vi "benchmarks_fileSHA1.vi"() -> ()   [LabVIEW 2013]
uses:
  SHA-1/SHA-1.lvclass
  <vilib>/Analysis/baseanly.llb/Mean (DBL).vi
  SHA-1/Enqueue File.vi
  SHA-1/pad.vi
  <vilib>/Analysis/NI_AALBase.lvlib
  SHA-1/SHA-1.lvlib
panel:
  out "MISSING ALGORITHM":bool
  out "equal hashes":bool
  out "% gain":dbl
  out "LVOS":dbl
  out "Other Algo":dbl
  in  "filepath":path
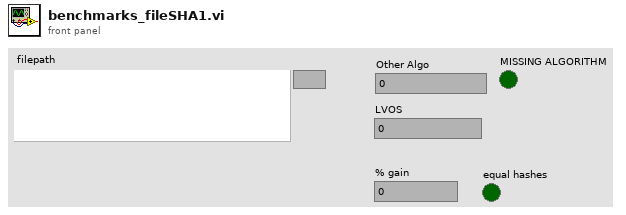
[diagram p1: front panel]
types:
  T1 = enum16{"open", "replace", "create", "open or create", "replace or create", "replace or create with confirmation"}
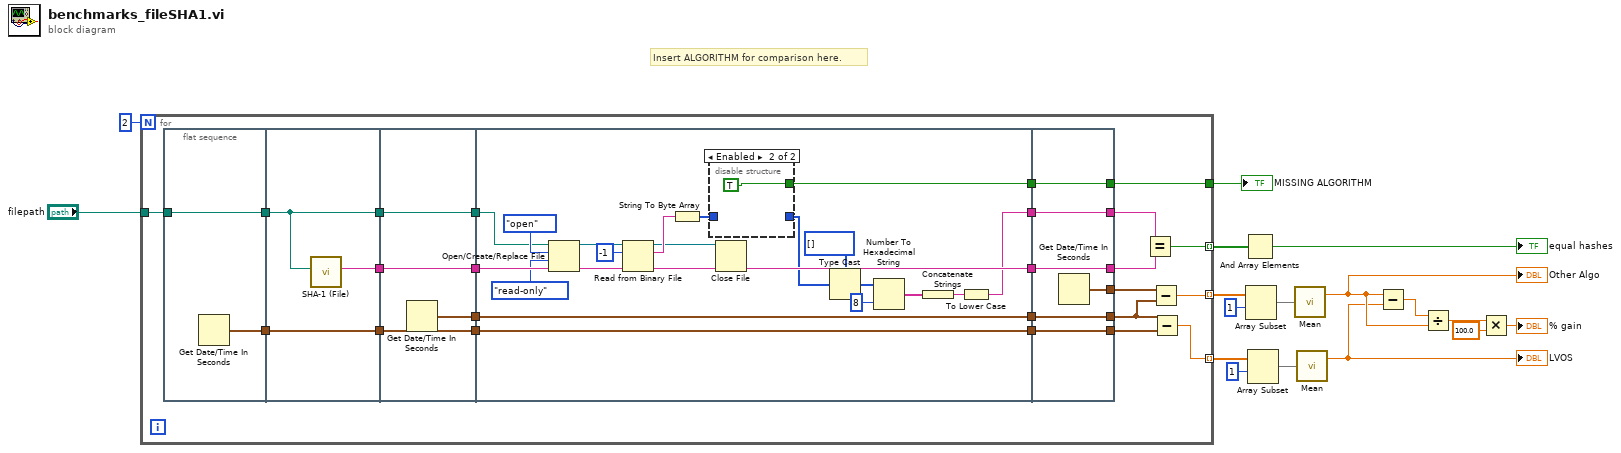
[diagram p0: block diagram]
diagram:
  # "Insert ALGORITHM for comparison here."
  n1 = for {
    N: 2 -> [_]
    tunnel: "filepath" -> [w28]
    tunnel: [w22] -> w16 mode=indexing
    tunnel: [w21] -> w9 mode=indexing
    tunnel: [w20] -> w8 mode=indexing
    tunnel: [w19] -> w1
    n2 = flat-sequence {
      tunnel: w28 -> [w43]
      tunnel: [w43] -> w41
      tunnel: [w42] -> w40
      tunnel: [w45] -> w39
      tunnel: w41 -> [w45]
      tunnel: w40 -> [w46]
      tunnel: [w46] -> w38
      tunnel: [w44] -> w37
      tunnel: w39 -> [w50]
      tunnel: [w50] -> w36
      tunnel: [w49] -> w35
      tunnel: [w48] -> w34
      tunnel: w38 -> [w48]
      tunnel: [w47] -> w33
      tunnel: w37 -> [w47]
      tunnel: w36 -> [w60]
      tunnel: [w71] -> w32
      tunnel: w35 -> [w71]
      tunnel: [w70] -> w31
      tunnel: w34 -> [w70]
      tunnel: [w54] -> w30
      tunnel: [w69] -> w29
      tunnel: w33 -> [w69]
      tunnel: [w51] -> w18
      tunnel: [w79] -> w26
      tunnel: w32 -> [w79]
      tunnel: [w78] -> w25
      tunnel: w31 -> [w78]
      tunnel: [w77] -> w27
      tunnel: [w76] -> w24
      tunnel: w30 -> [w76]
      tunnel: [w75] -> w23
      tunnel: w29 -> [w75]
      tunnel: [w74] -> w19
      tunnel: w18 -> [w74]
      frame #0 {
        n3 = Get Date/Time In Seconds() -> (seconds since 1Jan1904=w42:timestamp)
      }
      frame #1 {
        n4 = call "SHA-1 (File).vi"("filepath"=w45) -> ("SHA-1 hash"=w44:string)  [unwired: 10 in]
      }
      frame #2 {
        n5 = Get Date/Time In Seconds() -> (seconds since 1Jan1904=w49:timestamp)
      }
      frame #3 {
        n6 = Open/Create/Replace File(file path (use dialog)=w60, operation (0:open)=T1."open", access (0:read/write)=enum16{"read/write", "read-only", "write-only"}."read-only") -> (refnum out=w63:refnum<file>, error out=w64:errorcluster)  [unwired: 3 in, 1 out]
        n7 = Read from Binary File(8:w64, 10:-1 ("count (1)"), 11:w63) -> (0:w67:errorcluster, 2:w68:string, 3:w66:refnum<file>)  [unwired: 3 in, 1 out]
        n8 = String To Byte Array(string=w68) -> (unsigned byte array=w52:u8[])
        n9 = disable-structure shown="Enabled" {
          disable-tunnel: [w72 _] -> w53
          disable-tunnel: w52 -> [w72 _]
          disable-tunnel: [_ TRUE] -> w51
          frame Disabled {
          }
          frame Enabled {
          }
        }
        n10 = Close File(refnum=w66, error in=w67) -> ()  [unwired: 2 out]
        n11 = Type Cast(type=u32[] [] ("U32"), x=w53) -> (*(type *) &x=w57:u32[])
        n12 = Number To Hexadecimal String(1:i16 8 ("width (-)"), 2:w57) -> (0:w56:string[])
        n13 = Concatenate Strings(w56) -> (w55:string)
        n14 = To Lower Case(string=w55) -> (all lower case string=w54:string)
      }
      frame #4 {
        n15 = Get Date/Time In Seconds() -> (seconds since 1Jan1904=w77:timestamp)
      }
    }
    n16 = Equal?(x=w24, y=w23) -> (x = y?=w22:bool)
    n17 = Subtract(x=w27, y=w26) -> (x-y=w21:dbl)
    n18 = Subtract(x=w26, y=w25) -> (x-y=w20:dbl)
  }
  "MISSING ALGORITHM" <- w1
  n19 = And Array Elements(Boolean array=w16) -> (logical AND=→"equal hashes":bool)
  n20 = Array Subset(array=w9, index=1) -> (w12:dbl[])  [unwired: 1 in]
  n21 = Array Subset(array=w8, index=1) -> (w11:dbl[])  [unwired: 1 in]
  n22 = call-poly <vilib>:"Mean.vi"("X"=w12) -> ("mean"=w4:dbl)  [unwired: 1 out]
  "Other Algo" <- w4
  n23 = call-poly <vilib>:"Mean.vi"("X"=w11) -> ("mean"=w3:dbl)  [unwired: 1 out]
  "LVOS" <- w3
  n24 = Subtract(x=w4, y=w3) -> (x-y=w7:dbl)
  n25 = Divide(x=w7, y=w4) -> (x/y=w5:dbl)
  n26 = Multiply(x=w5, y=100.0) -> (x*y=→"% gain":dbl)
